vi "PrepareWaveformDataForTDMS.vi"(8 "error in (no error)":errorcluster, 11 "WaveformArray in":waveform(dbl)[](array[waveform])) -> (0 "error out":errorcluster, 1 "Measurement Data":dbl[][](array[numeric]), 2 "Channel Names":string[](array[string]))   [LabVIEW 2018, in "Visualization.lvlib" / "VisualizeSensor.lvclass"]
uses:
  VisualizeSensor.lvclass
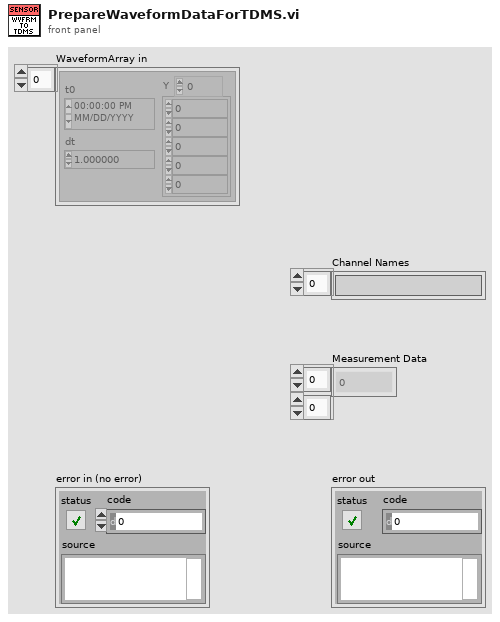
[diagram p1: front panel]
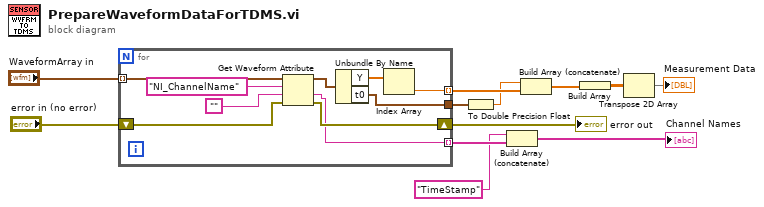
[diagram p0: block diagram]
diagram:
  n1 = for {
    tunnel: "WaveformArray in" -> [w22] mode=indexing
    tunnel: [w17] -> w11
    tunnel: [w16] -> w8 mode=indexing
    shift-right: [w14] -> w9
    shift-left: "error in (no error)" -> [w15]
    tunnel: [w13] -> w6 mode=indexing
    n2 = Get Waveform Attribute(4:w15, 5:"", 6:"NI_ChannelName" ("name"), 7:w22) -> (0:w14:errorcluster, 1:w13:string, 3:w19:waveform(dbl))  [unwired: 1 out]
    n3 = Unbundle By Name(w19) -> ("Y"=w18:dbl[], "t0"=w17:timestamp)
    n4 = Index Array(array=w18) -> (element=w16:dbl)  [unwired: 1 in]
  }
  "error out" <- w9
  n5 = To Double Precision Float(number=w11) -> (double precision float=w7:dbl)
  n6 = Build Array (concatenate)("TimeStamp" ("name"), w6) -> (→"Channel Names":string[])
  n7 = Build Array (concatenate)(w7, w8) -> (w3:dbl[])
  n8 = Build Array(w3) -> (w2:dbl[][])
  n9 = Transpose 2D Array(2D array=w2) -> (transposed array=→"Measurement Data":dbl[][])
